vi "DAQMan Read Error Log File.vi"(8 "error in (no error)":errorcluster) -> (0 "error out":errorcluster, 2 "all rows":string[][](array[string]), 3 "Number of Rows":u32)   [LabVIEW 2012, in "Configuration Grandmaster.lvlib" / "Cfg Grandmaster.lvclass"]
uses:
  Classes/Cfg Grandmaster/Class Cfg Grandmaster/Cfg Grandmaster.lvclass
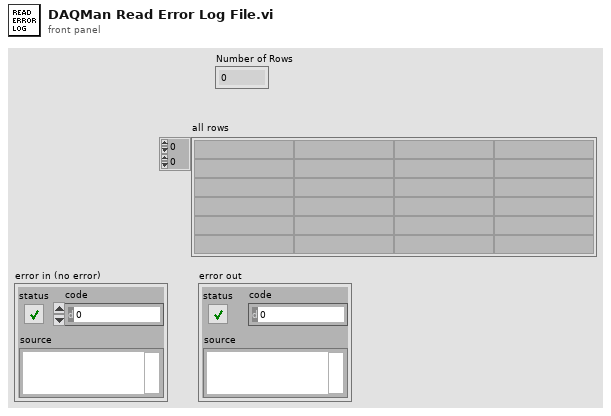
[diagram p1: front panel]
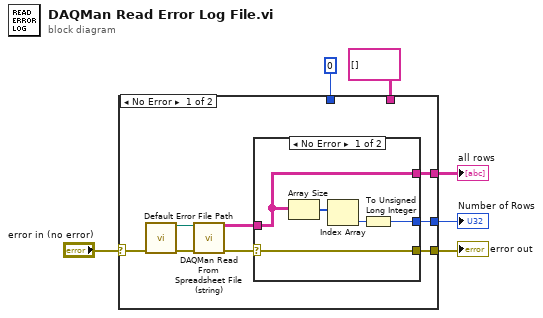
[diagram p0: block diagram]
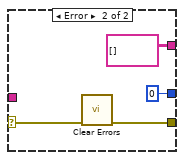
[diagram p2: hidden frame]
diagram:
  n1 = case shown="No Error" "error in (no error)" {
    selector: "error in (no error)" -> [w7 w26]
    tunnel: [w14 w24] -> w6
    tunnel: [w9 w26] -> w5
    tunnel: [w8 w25] -> w4
    tunnel: string[][] [] ("all rows") -> [_ w25]
    tunnel: u32 0 -> [_ w24]
    frame No Error {
      n2 = call "Default Error File Path.vi"("error in (no error)"=w7) -> ("error out"=w12:errorcluster, "Default Path"=w13:path)  [unwired: 9 in]
      n3 = call "DAQMan Read From Spreadsheet File (string).vi"("file path (dialog if empty)"=w13, "error in"=w12) -> ("all rows"=w11:string[][], "error out"=w10:errorcluster)  [unwired: 8 in, 4 out]
      n4 = case shown="No Error" w10 {
        selector: w10 -> [w16 w21]
        tunnel: [w19 u32 0] -> w14
        tunnel: w11 -> [w15 _]
        tunnel: [w16 w20] -> w9
        tunnel: [w15 string[][] [] ("all rows")] -> w8
        frame No Error {
          n5 = Array Size(array=w15) -> (size(s)=w18:i32[])
          n6 = Index Array(array=w18) -> (element=w17:i32)  [unwired: 1 in]
          n7 = To Unsigned Long Integer(number=w17) -> (unsigned 32bit integer=w19:u32)
        }
        frame Error {
          n8 = call <vilib>:"Clear Errors.vi"("error in (no error)"=w21) -> ("error out"=w20:errorcluster)  [unwired: 6 in]
        }
      }
    }
    frame Error {
    }
  }
  "Number of Rows" <- w6
  "error out" <- w5
  "all rows" <- w4
